vi "Save To Panel Layout File.vi"(5 "include size in file name? (F)":bool, 7 "panel layout folder (\"\")":path, 8 "error in":errorcluster, 9 "layout keyword (\"\")":string, 10 "VI path":path, 11 "panel layout in":refnum<class "VI Panel Layout.lvclass">) -> (0 "error out":errorcluster, 1 "saved?":bool, 3 "panel layout out":refnum<class "VI Panel Layout.lvclass">)   [LabVIEW 2012, in "NI_SE_Front Panel Layout.lvlib" / "VI Panel Layout.lvclass"]
doc: "Save the panel layout description to disk.\n\nIf <b>panel layout folder</b> is wired, the file will be saved in that folder. Otherwise, it will be saved next to the VI specified in <b>VI path</b>.\n\nIf <b>layout keyword</b> is wired, the keyword will be included in the file name."
uses:
  VI Panel Layout.lvclass
  VI Panel Layout.lvclass/VI Panel Layout.ctl
  <vilib>/Utility/libraryn.llb/Check if File or Folder Exists.vi
  NI_SE_Front Panel Layout.lvlib
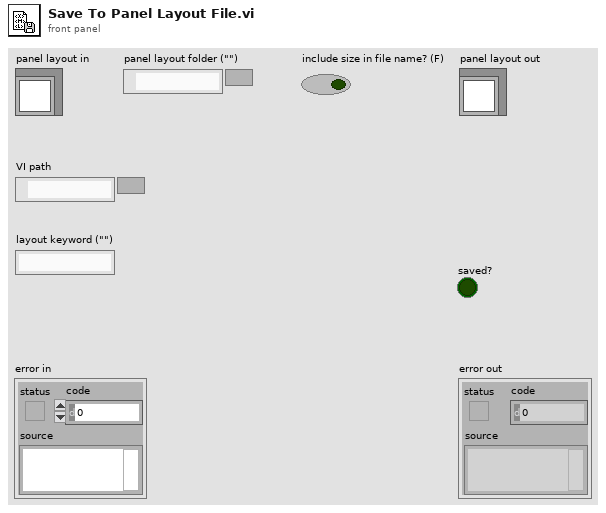
[diagram p1: front panel]
types:
  T1 = enum16{"open", "replace", "create", "open or create", "replace or create", "replace or create with confirmation"}
  T2 = typedef "LVRectTypeDef.ctl" = cluster{"Left":i16, "Top":i16, "Right":i16, "Bottom":i16}
  T3 = typedef "LVPointTypeDef.ctl" = cluster{"Horizontal":i16, "Vertical":i16}
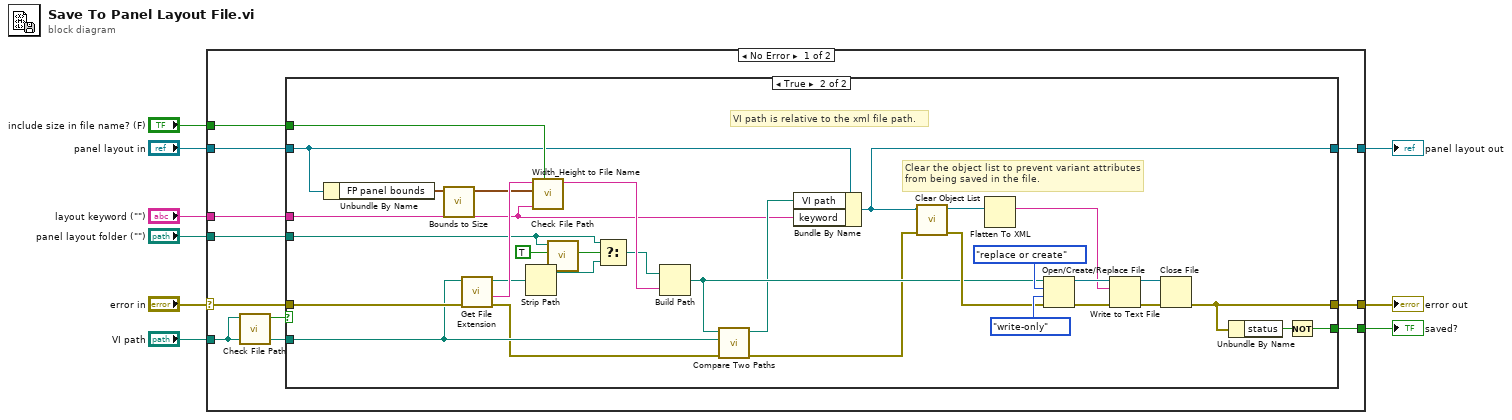
[diagram p0: block diagram]
diagram:
  n1 = case shown="No Error" "error in" {
    selector: "error in" -> [w19 w55]
    tunnel: [w18 w55] -> w8
    tunnel: [w16 w54] -> w6
    tunnel: "panel layout in" -> [w17 w54]
    tunnel: "VI path" -> [w12 _]
    tunnel: "layout keyword (\"\")" -> [w15 _]
    tunnel: [w14 _] -> w3
    tunnel: "panel layout folder (\"\")" -> [w13 _]
    tunnel: "include size in file name? (F)" -> [w10 _]
    frame No Error {
      n2 = call "Check File Path.vi"("path"=w12) -> ("valid path?"=w11:bool)  [unwired: 9 in, 1 out]
      n3 = case shown="True" w11 {
        tunnel: w19 -> [w20 w38]
        tunnel: [w20 w40] -> w18
        tunnel: w17 -> [w21 w25]
        tunnel: w12 -> [_ w28]
        tunnel: [w21 w22] -> w16
        tunnel: w15 -> [_ w23]
        tunnel: [_ w39] -> w14
        tunnel: w13 -> [_ w33]
        tunnel: w10 -> [_ w31]
        frame False {
        }
        frame True {
          # "VI path is relative to the xml file path."
          # "Clear the object list to prevent variant attributes from being saved in the file."
          n4 = Unbundle By Name(w25) -> ("FP panel bounds"=w44:T2)
          n5 = call "Bounds to Size.vi"("bounds"=w44) -> ("size"=w30:T3)  [unwired: 10 in]
          n6 = call <vilib>:"Get File Extension.vi"("error in (no error)"=w38, "file"=w28) -> ("error out"=w27:errorcluster, "filename without extension"=w43:string, "dup file"=w42:path)  [unwired: 6 in, 1 out]
          n7 = Strip Path(path=w42) -> (stripped path=w34:path)  [unwired: 1 out]
          n8 = call "Width_Height to File Name.vi"("include size in file name?"=w31, "keyword (\"\")"=w23, "size"=w30, "VI file name (no extension)"=w43) -> ("file name"=w41:string)  [unwired: 7 in]
          n9 = call "Check File Path.vi"("check if path exists? (F)"=TRUE, "path"=w33) -> ("path exists?"=w36:bool)  [unwired: 8 in, 1 out]
          n10 = Select(t=w33, s=w36, f=w34) -> (s? t:f=w37:path)
          n11 = Build Path(base path=w37, name or relative path=w41) -> (appended path=w29:path)
          n12 = call <vilib>:"Compare Two Paths.vi"("error in (no error)"=w27, "Path 2"=w28, "Path 1"=w29) -> ("error out"=w26:errorcluster, "Relative Path from 1 to 2"=w24:path)  [unwired: 5 in, 2 out]
          n13 = Bundle By Name(cluster=w25, "VI path"=w24, "keyword"=w23) -> (w22:refnum<class "VI Panel Layout.lvclass">)
          n14 = call "Clear Object List.vi"("error in (no error)"=w26, "VI Panel Layout in"=w22) -> ("error out"=w45:errorcluster, "VI Panel Layout out"=w46:refnum<class "VI Panel Layout.lvclass">)  [unwired: 8 in]
          n15 = Flatten To XML(anything=w46) -> (xml string=w47:string)
          n16 = Open/Create/Replace File(file path (use dialog)=w29, error in=w45, operation (0:open)=T1."replace or create", access (0:read/write)=enum16{"read/write", "read-only", "write-only"}."write-only") -> (refnum out=w49:refnum<file>, error out=w48:errorcluster)  [unwired: 2 in, 1 out]
          n17 = Write to Text File(file (use dialog)=w49, text=w47, error in=w48) -> (refnum out=w50:refnum<file>, error out=w51:errorcluster)  [unwired: 1 in, 1 out]
          n18 = Close File(refnum=w50, error in=w51) -> (error out=w40:errorcluster)  [unwired: 1 out]
          n19 = Unbundle By Name(w40) -> ("status"=w32:bool)
          n20 = Not(x=w32) -> (.not. x?=w39:bool)
        }
      }
    }
    frame Error {
    }
  }
  "error out" <- w8
  "panel layout out" <- w6
  "saved?" <- w3
